vi "RemoveVirtual.vi"(8 "error in (no error)":errorcluster, 11 "Project.lvclass In":refnum<class "Project.lvclass">) -> (0 "error out":errorcluster, 2 "VirtualIdx":i32=-1, 3 "Project.lvclass Out":refnum<class "Project.lvclass">)   [LabVIEW 2014, in "Project.lvclass"]
uses:
  Project.lvclass
  VirtualSetupDataTypeDefine.ctl
  Virtual/Control/AllVirtualTypeData.ctl
  Project.lvclass/Project.ctl
  Virtual/VirtualOrigin.lvclass
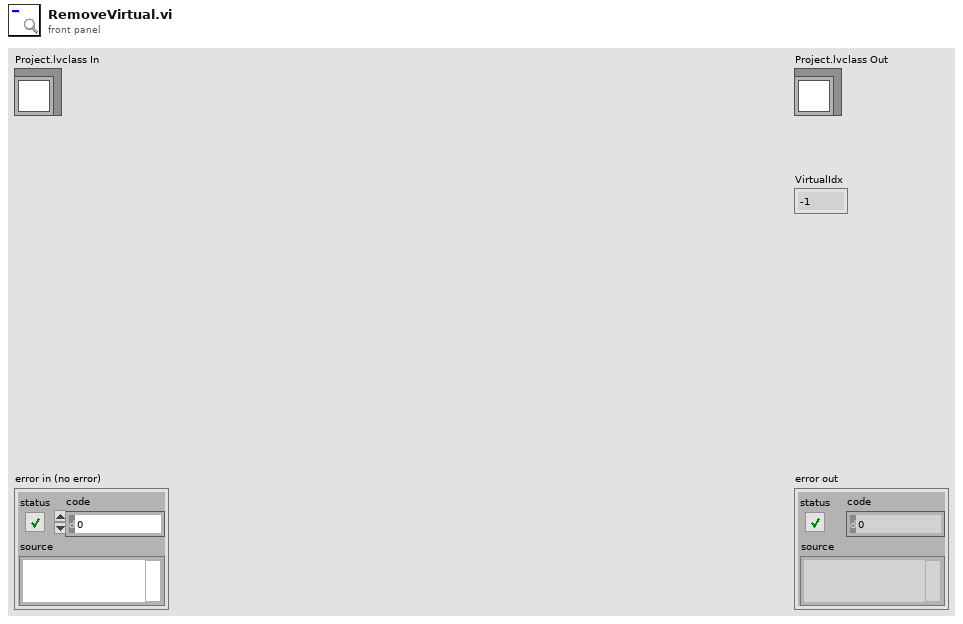
[diagram p1: front panel]
types:
  T1 = typedef "Project.lvclass/VirtualSetupDataTypeDefine.ctl" = T2[]
  T2 = typedef "VirtualOrigin.lvclass/AllVirtualTypeData.ctl" = cluster{"Search Name":string, "Start X":dbl, "Increase X":dbl, "X Step":i32, "Start Y":dbl, "Increase Y":dbl, "Y Step":i32, "Sensor":i32}
  T3 = typedef "Project.lvclass/ProjectDataTableTypeDefine.ctl" = string[][]
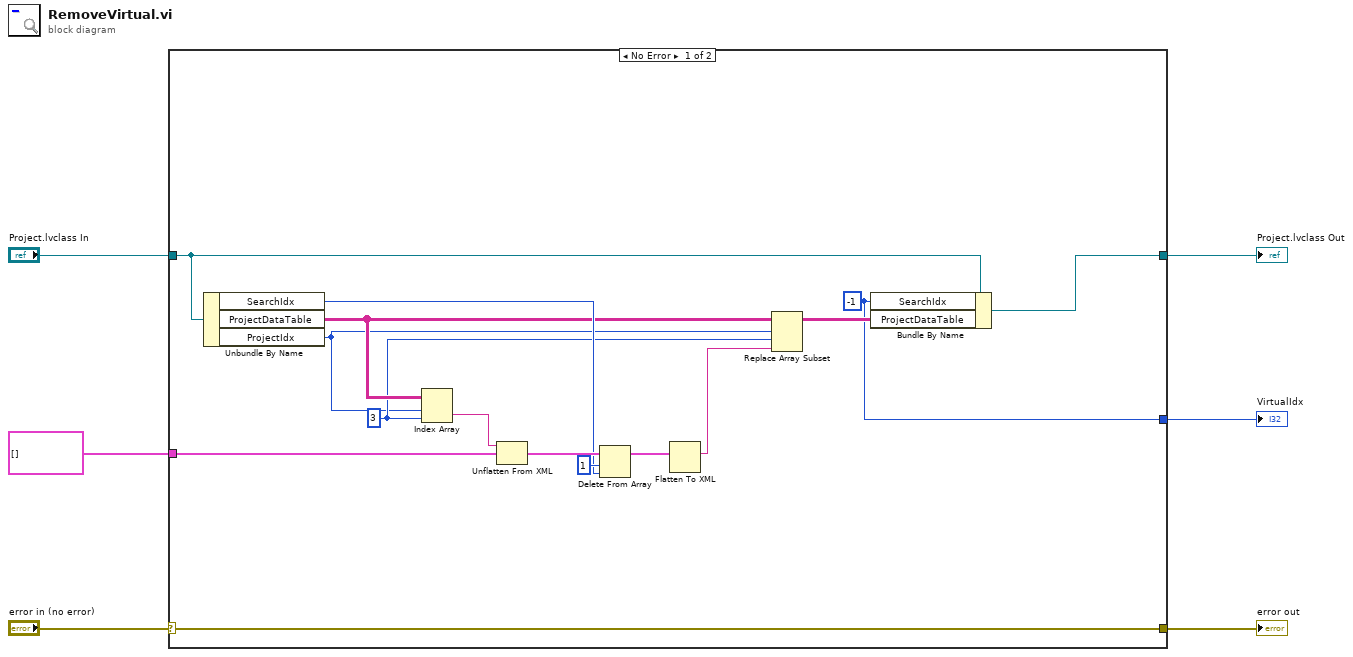
[diagram p0: block diagram]
diagram:
  n1 = case shown="No Error" "error in (no error)" {
    selector: "error in (no error)" -> [w21 w23]
    tunnel: [w21 w23] -> w5
    tunnel: "Project.lvclass In" -> [w20 w22]
    tunnel: [w19 w22] -> w3
    tunnel: [w8 _] -> w2
    tunnel: T1 [] ("VirtualSetupClusterArray") -> [w7 _]
    frame No Error {
      w8 = -1 ("StepIdx")
      w12 = 3 ("disabled index (col)")
      n2 = Unbundle By Name(w20) -> ("SearchIdx"=w15:i32, "ProjectDataTable"=w13:T3, "ProjectIdx"=w11:i32)
      n3 = Index Array(array=w13, index (row)=w11, index (col)=w12) -> (element=w18:string)
      n4 = Unflatten From XML(xml string=w18, type=w7) -> (value=w17:T1)  [unwired: 1 in, 1 out]
      n5 = Delete From Array(array=w17, length=1, index=w15) -> (array with subset deleted=w14:T1)  [unwired: 1 out]
      n6 = Flatten To XML(anything=w14) -> (xml string=w10:string)
      n7 = Replace Array Subset(array=w13, new element=w10, index (row)=w11, index (col)=w12) -> (w9:T3)
      n8 = Bundle By Name(cluster=w20, "SearchIdx"=w8, "ProjectDataTable"=w9) -> (w19:refnum<class "Project.lvclass">)
    }
    frame Error {
    }
  }
  "error out" <- w5
  "Project.lvclass Out" <- w3
  "VirtualIdx" <- w2
